vi "Battery Level Control.vi"(9 "Power Level":u8, 10 "Battery Power ref":refnum<vi>) -> ()   [LabVIEW 2025]
uses:
  Ctrls/Battery Control.ctl
  <vilib>/Utility/miscctls.llb/LVForegroundBackgroundColorsTypeDef.ctl
panel:
  out "Battery Power":T1 scale=0.0..100.0
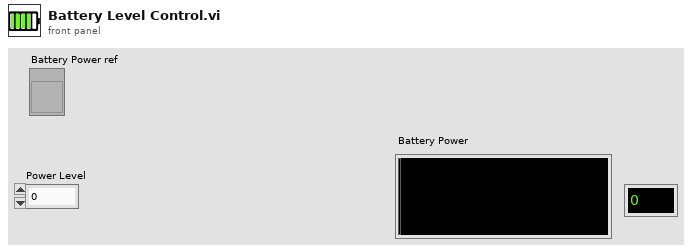
[diagram p1: front panel]
types:
  T1 = typedef "Battery Control.ctl" = u8
  T2 = typedef "LVForegroundBackgroundColorsTypeDef.ctl" = cluster{"Foreground Color":u32, "Background Color":u32}
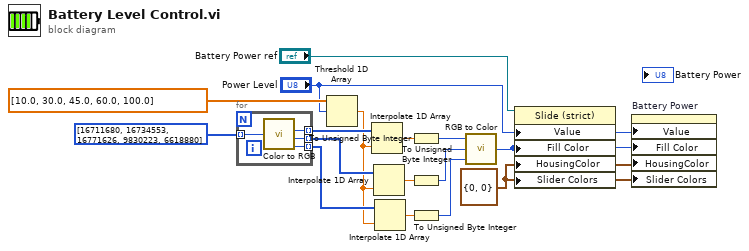
[diagram p0: block diagram]
diagram:
  w1 = T2 {"Foreground Color"=0, "Background Color"=0} ("Slider Colors")
  n1 = for {
    tunnel: [w20] -> w12 mode=indexing
    tunnel: [w19] -> w13 mode=indexing
    tunnel: [w18] -> w14 mode=indexing
    tunnel: u32[] [16711680, 16734553, 16771626, 9830223, 6618880] ("Colors") -> [w17] mode=indexing
    n2 = call <vilib>:"Color to RGB.vi"("Color"=w17) -> ("R"=w20:u8, "G"=w19:u8, "B"=w18:u8)  [unwired: 1 out]
  }
  n3 = Threshold 1D Array(2:"Power Level", 3:dbl[] [10.0, 30.0, 45.0, 60.0, 100.0] ("Values")) -> (0:w11:dbl)  [unwired: 1 in]
  n4 = Interpolate 1D Array(1:w11, 2:w12) -> (0:w10:dbl)
  n5 = Interpolate 1D Array(1:w11, 2:w13) -> (0:w9:dbl)
  n6 = Interpolate 1D Array(1:w11, 2:w14) -> (0:w8:dbl)
  n7 = To Unsigned Byte Integer(number=w10) -> (unsigned 8bit integer=w7:u8)
  n8 = To Unsigned Byte Integer(number=w9) -> (unsigned 8bit integer=w6:u8)
  n9 = To Unsigned Byte Integer(number=w8) -> (unsigned 8bit integer=w5:u8)
  n10 = call <vilib>:"RGB to Color.vi"("B"=w5, "G"=w6, "R"=w7) -> ("Color"=w2:u32)
  n11 = property class="Slide (strict)"(reference="Battery Power ref", "Value"="Power Level", "Fill Color"=w2, "HousingColor"=w1, "Slider Colors"=w1) -> ()  [unwired: 1 in, 2 out]
  n12 = property on="Battery Power" class="Slide (strict)"("Value"="Power Level", "Fill Color"=w2, "HousingColor"=w1, "Slider Colors"=w1) -> ()  [unwired: 2 in, 2 out]
